vi "Open DAQ Racks.vi"(10 "DAQ Rack Path":path) -> (3 "DAQ Rack Refs":refnum<vi>[](array[refnum]))   [LabVIEW 2019]
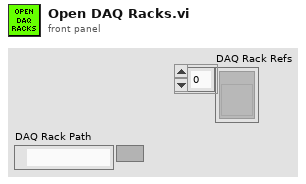
[diagram p1: front panel]
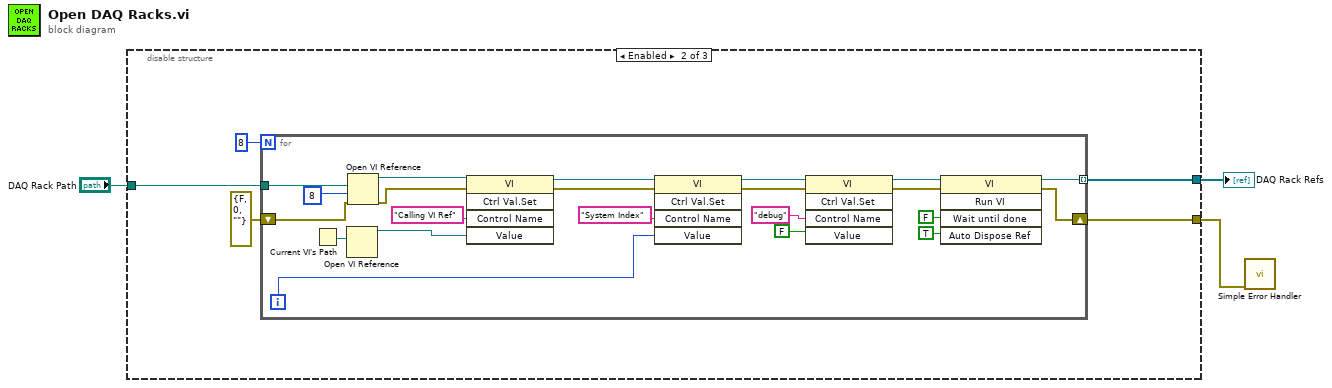
[diagram p0: block diagram]
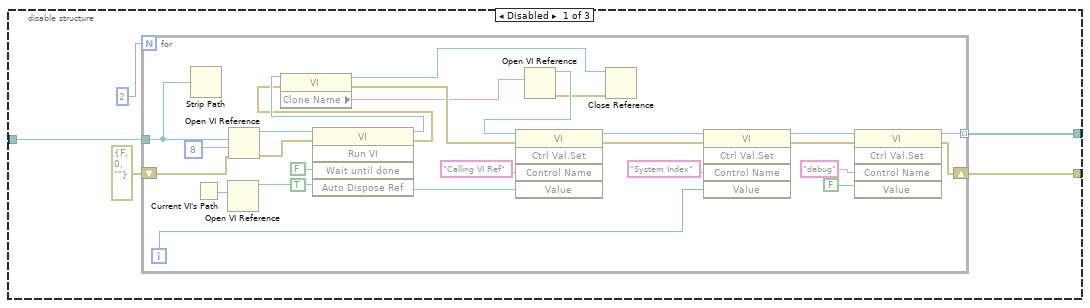
[diagram p2: hidden frame]
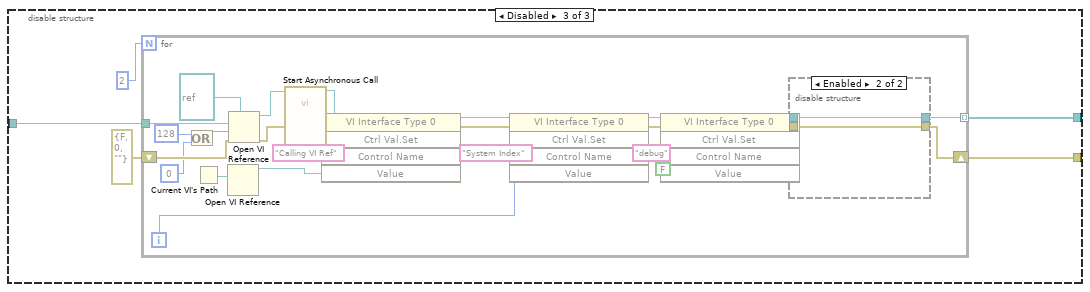
[diagram p3: hidden frame]
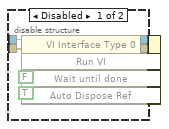
[diagram p4: hidden frame]
diagram:
  n1 = disable-structure shown="Enabled" {
    disable-tunnel: "DAQ Rack Path" -> [w8 w40 w67]
    disable-tunnel: [w7 w39 w66] -> w2
    disable-tunnel: [w4 w36 w63] -> w1
    frame Disabled {
      n2 = for {
        N: 2 -> [_]
        tunnel: w8 -> [w12]
        tunnel: [w14] -> w7 mode=indexing
        shift-right: [w13] -> w4
        shift-left: errorcluster {"status"=FALSE, "code"=0, "source"=""} ("error out") -> [w24]
        i -> [w27]
        n3 = Strip Path(path=w12) -> ()  [unwired: 2 out]
        n4 = Current VI's Path() -> (path=w32:path)
        n5 = Open VI Reference(vi path=w32) -> (vi reference=w31:refnum<vi>)  [unwired: 5 in, 1 out]
        n6 = Open VI Reference(vi path=w12, options=8, error in (no error)=w24) -> (vi reference=w19:refnum<vi>, error out=w17:errorcluster)  [unwired: 3 in]
        n7 = invoke class="VI" method="Run VI"(reference=w19, error in=w17, "Wait until done"=FALSE ("Wait Until Done"), "Auto Dispose Ref"=TRUE ("Auto Dispose Reference")) -> (reference out=w18:refnum<vi>, error out=w16:errorcluster)  [unwired: 1 in, 3 out]
        n8 = property class="VI"(reference=w18, error in=w16) -> (reference out=w10:refnum<vi>, error out=w15:errorcluster, "Clone Name"=w11:string)
        n9 = Open VI Reference(vi path=w11) -> (vi reference=w22:refnum<vi>, error out=w9:errorcluster)  [unwired: 5 in]
        n10 = invoke class="VI" method="Ctrl Val.Set"(reference=w22, error in=w15, "Control Name"="Calling VI Ref", "Value"=w31) -> (reference out=w29:refnum<vi>, error out=w26:errorcluster)  [unwired: 1 in, 3 out]
        n11 = Close Reference(reference=w10, error in (no error)=w9) -> ()  [unwired: 1 out]
        n12 = invoke class="VI" method="Ctrl Val.Set"(reference=w29, error in=w26, "Control Name"="System Index", "Value"=w27) -> (reference out=w28:refnum<vi>, error out=w25:errorcluster)  [unwired: 1 in, 3 out]
        n13 = invoke class="VI" method="Ctrl Val.Set"(reference=w28, error in=w25, "Control Name"="debug", "Value"=FALSE ("Wait Until Done")) -> (reference out=w14:refnum<vi>, error out=w13:errorcluster)  [unwired: 1 in, 3 out]
      }
    }
    frame Enabled {
      n14 = for {
        N: 8 -> [_]
        tunnel: w40 -> [w62]
        tunnel: [w61] -> w39 mode=indexing
        shift-right: [w44] -> w36
        shift-left: errorcluster {"status"=FALSE, "code"=0, "source"=""} ("error out") -> [w43]
        i -> [w49]
        n15 = Current VI's Path() -> (path=w55:path)
        n16 = Open VI Reference(vi path=w55) -> (vi reference=w54:refnum<vi>)  [unwired: 5 in, 1 out]
        n17 = Open VI Reference(vi path=w62, options=8, error in (no error)=w43) -> (vi reference=w42:refnum<vi>, error out=w48:errorcluster)  [unwired: 3 in]
        n18 = invoke class="VI" method="Ctrl Val.Set"(reference=w42, error in=w48, "Control Name"="Calling VI Ref", "Value"=w54) -> (reference out=w51:refnum<vi>, error out=w47:errorcluster)  [unwired: 1 in, 3 out]
        n19 = invoke class="VI" method="Ctrl Val.Set"(reference=w51, error in=w47, "Control Name"="System Index", "Value"=w49) -> (reference out=w50:refnum<vi>, error out=w46:errorcluster)  [unwired: 1 in, 3 out]
        n20 = invoke class="VI" method="Ctrl Val.Set"(reference=w50, error in=w46, "Control Name"="debug", "Value"=FALSE ("Wait Until Done")) -> (reference out=w53:refnum<vi>, error out=w45:errorcluster)  [unwired: 1 in, 3 out]
        n21 = invoke class="VI" method="Run VI"(reference=w53, error in=w45, "Wait until done"=FALSE ("Wait Until Done"), "Auto Dispose Ref"=TRUE ("Auto Dispose Reference")) -> (reference out=w61:refnum<vi>, error out=w44:errorcluster)  [unwired: 1 in, 3 out]
      }
    }
    frame Disabled {
      n22 = for {
        N: 2 -> [_]
        tunnel: w67 -> [w73]
        tunnel: [w91] -> w66 mode=indexing
        shift-right: [w77] -> w63
        shift-left: errorcluster {"status"=FALSE, "code"=0, "source"=""} ("error out") -> [w76]
        i -> [w82]
        n23 = Or(x=128 ("options"), y=0 ("options")) -> (x .or. y?=w70:i32)
        n24 = Current VI's Path() -> (path=w87:path)
        n25 = Open VI Reference(vi path=w87) -> (vi reference=w86:refnum<vi>)  [unwired: 5 in, 1 out]
        n26 = Open VI Reference(type specifier VI Refnum (for type only)=refnum<vi> refnum ("reference"), vi path=w73, options=w70, error in (no error)=w76) -> (vi reference=w75:refnum<vi>, error out=w81:errorcluster)  [unwired: 2 in]
        n27 = call-by-ref "Start Asynchronous Call"(reference=w75) -> (reference out=w69:refnum<vi>)  [unwired: 13 in, 1 out]
        n28 = invoke class="VI Interface Type 0" method="Ctrl Val.Set"(reference=w69, error in=w81, "Control Name"="Calling VI Ref", "Value"=w86) -> (reference out=w84:refnum<vi>, error out=w80:errorcluster)  [unwired: 1 in, 3 out]
        n29 = invoke class="VI Interface Type 0" method="Ctrl Val.Set"(reference=w84, error in=w80, "Control Name"="System Index", "Value"=w82) -> (reference out=w83:refnum<vi>, error out=w79:errorcluster)  [unwired: 1 in, 3 out]
        n30 = invoke class="VI Interface Type 0" method="Ctrl Val.Set"(reference=w83, error in=w79, "Control Name"="debug", "Value"=FALSE ("Wait Until Done")) -> (reference out=w68:refnum<vi>, error out=w78:errorcluster)  [unwired: 1 in, 3 out]
        n31 = disable-structure shown="Enabled" {
          disable-tunnel: [w97 w99] -> w91
          disable-tunnel: w68 -> [w96 w99]
          disable-tunnel: w78 -> [w95 w98]
          disable-tunnel: [w94 w98] -> w77
          frame Disabled {
            n32 = invoke class="VI Interface Type 0" method="Run VI"(reference=w96, error in=w95, "Wait until done"=FALSE ("Wait Until Done"), "Auto Dispose Ref"=TRUE ("Auto Dispose Reference")) -> (reference out=w97:refnum<vi>, error out=w94:errorcluster)  [unwired: 1 in, 3 out]
          }
          frame Enabled {
          }
        }
      }
    }
  }
  "DAQ Rack Refs" <- w2
  n33 = call <vilib>:"Simple Error Handler.vi"("error in (no error)"=w1) -> ()  [unwired: 4 in, 5 out]
